vi "ADC (A).vi"(0 "Adc":refnum<k24>, 1 "Loops 2":i32, 2 "Gain":i32(ring) items=["Gain_1"=0, "Gain_10"=64, "Gain_100"=128, "Gain_1000"=192], 3 "Loops":i32, 5 "Sampler Type":T1(ring), 7 "Gain 2":i32(ring) items=["Gain_1"=0, "Gain_10"=64, "Gain_100"=128, "Gain_1000"=192], 9 "usPerLoop 2":u16, 11 "error in":errorcluster, 12 "Channel":i32(ring) items=["16"=15, "15"=14, "14"=13, "13"=12, "12"=11, "11"=10, "10"=9, "9"=8, "8"=7, "7"=6, "6"=5, "5"=4, "4"=3, "3"=2, "2"=1, "1"=0], 13 "usPerLoop":u16) -> (4 "Sample":dbl, 6 "Disable MeanGain":u8, 8 "Disable MeanFixed":u8, 10 "Disable OneFixed":u8, 15 "error out":errorcluster)   [LabVIEW 2011]
doc: "Control the Analog/Digital Converter manually (advanced version)."
uses:
  C:/Program Files/Metrohm Autolab/Autolab SDK 1.10/EcoChemie.Autolab.Sdk.dll
  EcoChemie.Autolab.Sdk.dll
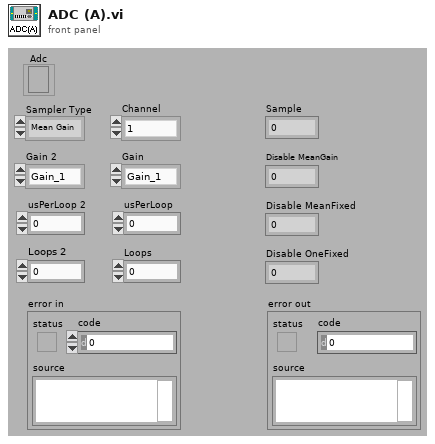
[diagram p1: front panel]
types:
  T1 = enum16{"Mean Gain", "Mean Fixed", "One Fixed", "One Gain"}
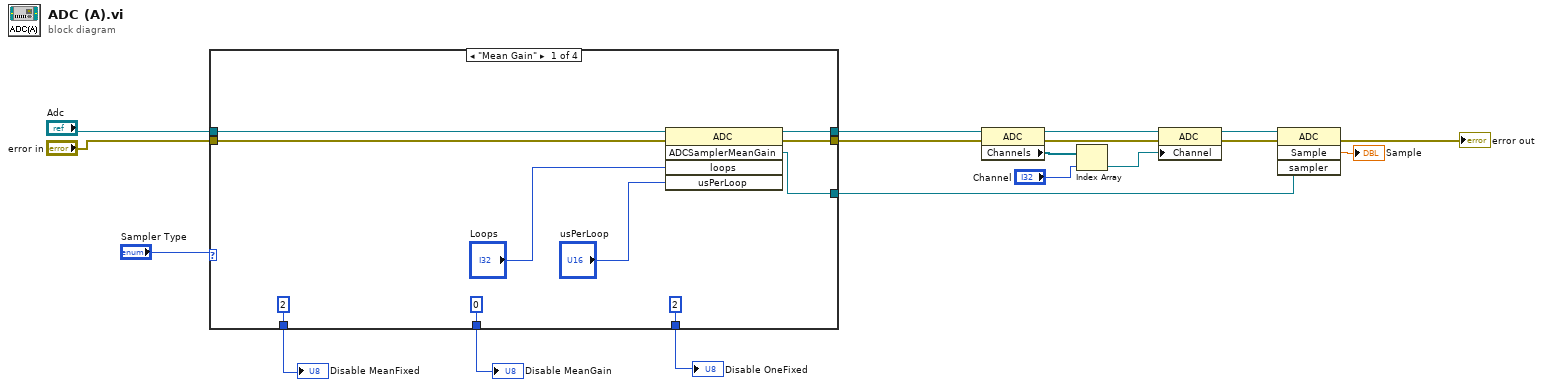
[diagram p0: block diagram]
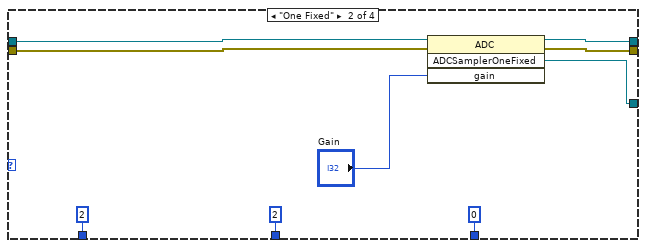
[diagram p2: hidden frame]
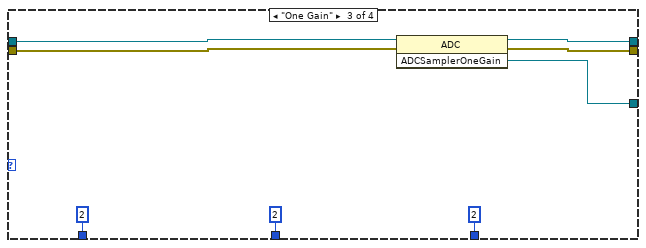
[diagram p3: hidden frame]
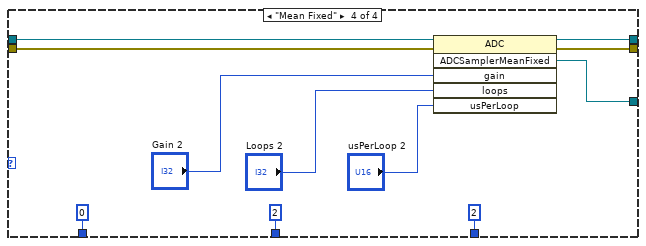
[diagram p4: hidden frame]
diagram:
  n1 = case shown="\"Mean Gain\"" "Sampler Type" {
    tunnel: [w25 w29 w45 w56] -> w1
    tunnel: [u8 2 ("Disabled") u8 2 ("Disabled") u8 2 ("Disabled") u8 0 ("Disabled")] -> w6
    tunnel: "Adc" -> [w28 w37 w44 w54]
    tunnel: [u8 2 ("Disabled") u8 0 ("Disabled") u8 2 ("Disabled") u8 2 ("Disabled")] -> w4
    tunnel: "error in" -> [w24 w34 w41 w52]
    tunnel: [w23 w33 w40 w51] -> w10
    tunnel: [w22 w32 w39 w50] -> w18
    tunnel: [u8 0 ("Disabled") u8 2 ("Disabled") u8 2 ("Disabled") u8 2 ("Disabled")] -> w5
    frame "Mean Gain" {
      n2 = invoke class="ADC" method="ADCSamplerMeanGain"(reference=w28, error in=w24, "loops"="Loops", "usPerLoop"="usPerLoop") -> (reference out=w22:refnum<k24>, error out=w23:errorcluster, "ADCSamplerMeanGain"=w25:refnum<k24>)  [unwired: 1 in, 2 out]
    }
    frame "One Fixed" {
      n3 = invoke class="ADC" method="ADCSamplerOneFixed"(reference=w37, error in=w34, "gain"="Gain") -> (reference out=w32:refnum<k24>, error out=w33:errorcluster, "ADCSamplerOneFixed"=w29:refnum<k24>)  [unwired: 1 in, 1 out]
    }
    frame "One Gain" {
      n4 = invoke class="ADC" method="ADCSamplerOneGain"(reference=w44, error in=w41) -> (reference out=w39:refnum<k24>, error out=w40:errorcluster, "ADCSamplerOneGain"=w45:refnum<k24>)  [unwired: 1 in]
    }
    frame "Mean Fixed" {
      n5 = invoke class="ADC" method="ADCSamplerMeanFixed"(reference=w54, error in=w52, "gain"="Gain 2", "loops"="Loops 2", "usPerLoop"="usPerLoop 2") -> (reference out=w50:refnum<k24>, error out=w51:errorcluster, "ADCSamplerMeanFixed"=w56:refnum<k24>)  [unwired: 1 in, 3 out]
    }
  }
  "Disable MeanFixed" <- w6
  "Disable MeanGain" <- w5
  "Disable OneFixed" <- w4
  n6 = property class="ADC"(reference=w18, error in=w10) -> (reference out=w17:refnum<k24>, error out=w16:errorcluster, "Channels"=w15:refnum<k24>[])
  n7 = Index Array(array=w15, index="Channel") -> (element=w14:refnum<k24>)
  n8 = property class="ADC"(reference=w17, error in=w16, "Channel"=w14) -> (reference out=w13:refnum<k24>, error out=w12:errorcluster)
  n9 = invoke class="ADC" method="Sample"(reference=w13, error in=w12, "sampler"=w1) -> (error out=→"error out":errorcluster, "Sample"=→"Sample":dbl)  [unwired: 1 in, 2 out]
